vi "Read Name.vi"(8 "error in":errorcluster, 11 "Custom Device Config in":refnum<class "Custom Device Config.lvclass">) -> (0 "error out":errorcluster, 2 "Name":string, 3 "Custom Device Config out":refnum<class "Custom Device Config.lvclass">)   [LabVIEW 2024, in "Parser.lvlib" / "Custom Device Config.lvclass"]
uses:
  Custom Device Config.lvclass
  Custom Device Config.lvclass/Custom Device Config.ctl
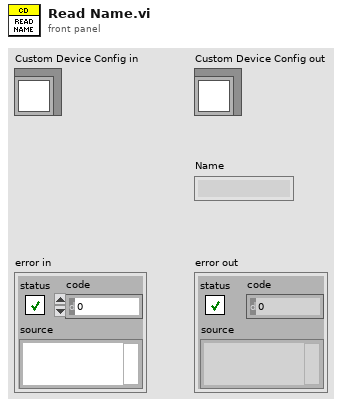
[diagram p1: front panel]
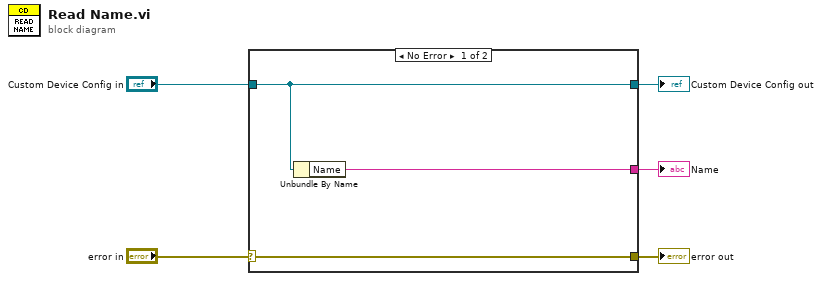
[diagram p0: block diagram]
diagram:
  n1 = case shown="No Error" "error in" {
    selector: "error in" -> [w8 w10]
    tunnel: [w8 w10] -> w4
    tunnel: [w7 w9] -> w2
    tunnel: "Custom Device Config in" -> [w7 w9]
    tunnel: [w6 _] -> w1
    frame No Error {
      n2 = Unbundle By Name(w7) -> ("Name"=w6:string)
    }
    frame Error {
    }
  }
  "error out" <- w4
  "Custom Device Config out" <- w2
  "Name" <- w1
